vi "AI test Drive Relays All v6.vi"(9 "Array #2":bool[](array[boolean]), 10 "Array #1":bool[](array[boolean]), 11 "Array #0":bool[](array[boolean])) -> (0 "error Array":errorcluster[](array[cluster]))   [LabVIEW 2013]
panel:
  # "LAB01-1 (START)"
  # "LAB02-1 (JIG)"
  # "LAB04-2 (START)"
  # "LAB01-1 (JIG)"
  # "LAB03-1 (START)"
  # "LAB04-2 (JIG)"
  # "LAB01-2 (START)"
  # "LAB05-1 (START)"
  # "LAB03-1 (JIG)"
  # "LAB01-2 (JIG)"
  # "LAB05-1 (JIG)"
  # "LAB03-2 (START)"
  # "LAB02-1 (START)"
  # "LAB05-2 (START)"
  # "LAB03-2 (JIG)"
  # "LAB05-2 (JIG)"
  # "LAB02-1 (JIG)"
  # "LAB04-1 (START)"
  # "LAB02-1 (START)"
  # "LAB04-1 (JIG)"
  # "RESET ALL"
  # "RESET TEMP"
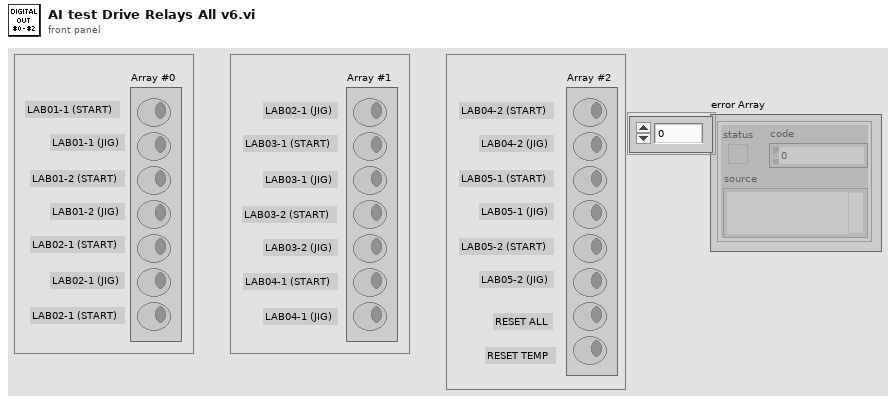
[diagram p1: front panel]
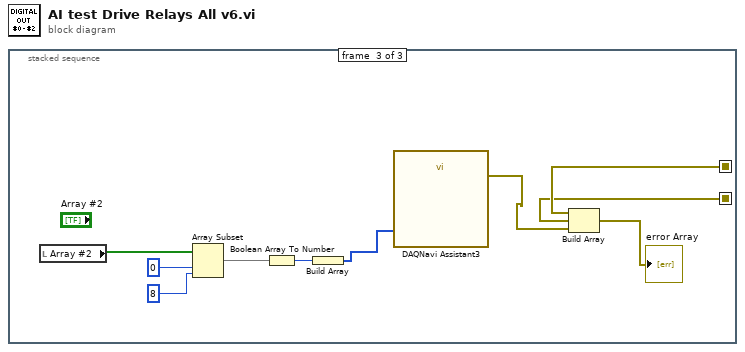
[diagram p0: block diagram]
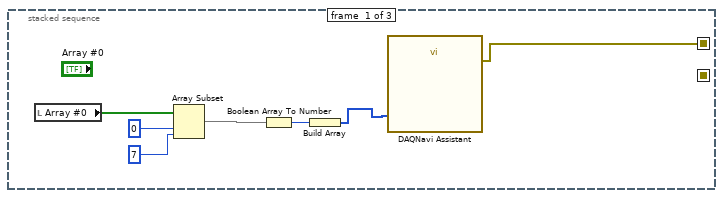
[diagram p2: hidden frame]
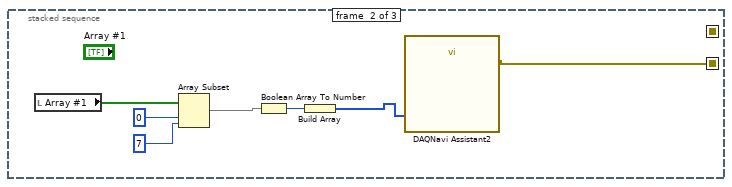
[diagram p3: hidden frame]
diagram:
  n1 = stacked-sequence {
    seq-local: [w1 _ _] -> [_ _ w19]
    seq-local: [_ w8 _] -> [_ _ w18]
    frame #0 {
      n2 = local read "Array #0"() -> (w6:bool[])
      n3 = Array Subset(array=w6, index=0, length=7) -> (w3:bool[])
      n4 = Boolean Array To Number(Boolean array=w3) -> (number=w7:u8)
      n5 = Build Array(w7) -> (w2:u8[])
      n6 = call "DAQNavi Assistant"("dataIn(U8Array)"=w2) -> ("error out"=w1:errorcluster)  [unwired: 26 in]
    }
    frame #1 {
      n7 = local read "Array #1"() -> (w11:bool[])
      n8 = Array Subset(array=w11, index=0, length=7) -> (w10:bool[])
      n9 = Boolean Array To Number(Boolean array=w10) -> (number=w14:u8)
      n10 = Build Array(w14) -> (w9:u8[])
      n11 = call "DAQNavi Assistant2"("dataIn(U8Array)"=w9) -> ("error out"=w8:errorcluster)  [unwired: 26 in]
    }
    frame #2 {
      n12 = local read "Array #2"() -> (w21:bool[])
      n13 = Array Subset(array=w21, index=0, length=8) -> (w20:bool[])
      n14 = Boolean Array To Number(Boolean array=w20) -> (number=w24:u8)
      n15 = Build Array(w24) -> (w16:u8[])
      n16 = call "DAQNavi Assistant3"("dataIn(U8Array)"=w16) -> ("error out"=w15:errorcluster)  [unwired: 26 in]
      n17 = Build Array(w19, w18, w15) -> (→"error Array":errorcluster[])
    }
  }
